vi "process_data.vi"(8 "Error in":errorcluster, 10 "JSON Payload":string, 11 "Data Cluster in":T1={"Status"="", "Data sources"=[], "Host name or address"="localhost", "Remote port"=35535, "Local port"=35535, "Key"="", "connection ID"=refnum, "Data Names"={""}}) -> (0 "Error out":errorcluster, 3 "Data Cluster out":T1={"Status"="", "Data sources"=[], "Host name or address"="localhost", "Remote port"=35535, "Local port"=35535, "Key"="", "connection ID"=refnum, "Data Names"={""}})   [LabVIEW 2014, in "get_data_mapper.lvlib"]
uses:
  get_data_mapper.lvlib
  Module Data--cluster.ctl
  C:/Github/get_data_mapping/Libraries/get_data_mapper/Encrypt.dll
  Encrypt.dll
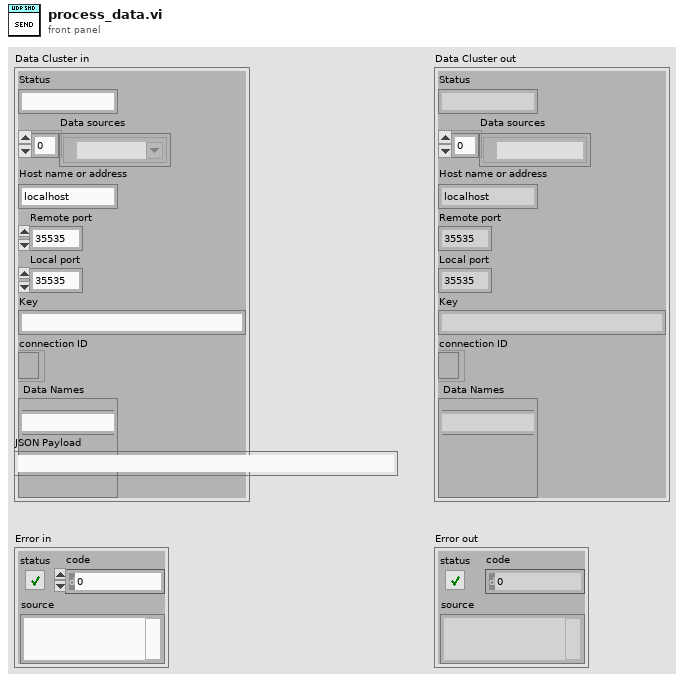
[diagram p1: front panel]
types:
  T1 = typedef "get_data_mapper.lvlib/Module Data--cluster.ctl" = cluster{"Status":string, "Data sources":refnum<k21>[], "Host name or address":string, "Remote port":u16, "Local port":u16, "Key":string, "connection ID":refnum<k16>, "Data Names":cluster{string}}
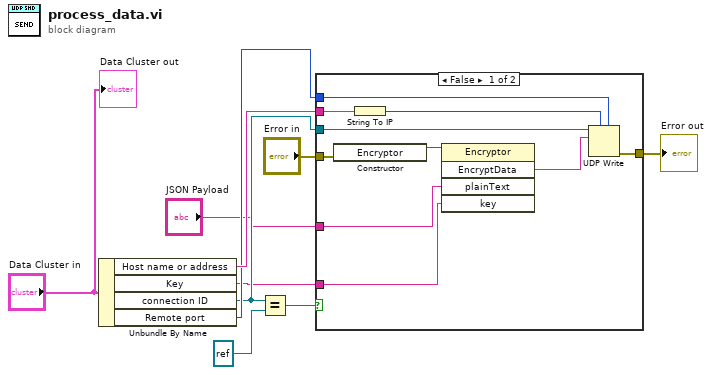
[diagram p0: block diagram]
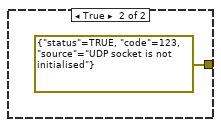
[diagram p2: hidden frame]
diagram:
  n1 = Unbundle By Name("Data Cluster in") -> ("Host name or address"=w7:string, "Key"=w3:string, "connection ID"=w5:refnum<k16>, "Remote port"=w6:u16)
  n2 = Equal?(x=w5, y=refnum<k16> refnum) -> (x = y?=w8:bool)
  n3 = case shown="False" w8 {
    tunnel: w7 -> [w19 _]
    tunnel: w6 -> [w18 _]
    tunnel: w5 -> [w17 _]
    tunnel: "JSON Payload" -> [w13 _]
    tunnel: w3 -> [w12 _]
    tunnel: "Error in" -> [w15 _]
    tunnel: [w16 errorcluster {"status"=TRUE, "code"=123, "source"="UDP socket is not initialised"} ("error out")] -> w1
    frame False {
      n4 = constructor class="Encryptor"(error in=w15) -> (reference out=w14:refnum<k24>)  [unwired: 2 in, 2 out]
      n5 = String To IP(1:w19) -> (0:w20:u32)
      n6 = invoke class="Encryptor" method="EncryptData"(reference=w14, "plainText"=w13, "key"=w12) -> ("EncryptData"=w11:string)  [unwired: 2 in, 4 out]
      n7 = UDP Write(address=w20, port or service name=w18, connection ID=w17, data in=w11) -> (error out=w16:errorcluster)  [unwired: 2 in, 1 out]
    }
    frame True {
    }
  }
  "Error out" <- w1
  "Data Cluster out" <- "Data Cluster in"
